vi "Index Texture.vi"(10 "Texture":T1, 11 "Point In Texture":T3) -> (3 "Colour":u32(colorbox))   [LabVIEW 2020, in "Raster (FPGA).lvlib"]
uses:
  Raster (FPGA).lvlib
  Point 2D (I32).ctl
  Texture.ctl
  Rectangle Dimensions.ctl
panel:
  in  "Use Texture (T)":bool=TRUE
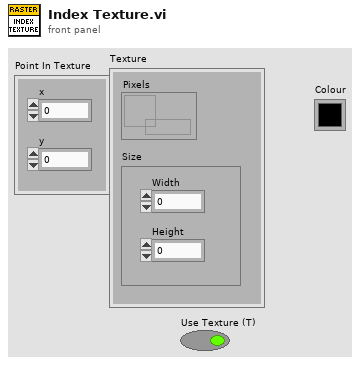
[diagram p1: front panel]
types:
  T1 = typedef "Raster (FPGA).lvlib/Texture.ctl" = cluster{"Pixels":refnum<data-value>, "Size":T2}
  T2 = typedef "Raster (FPGA).lvlib/Rectangle Dimensions.ctl" = cluster{"Width":u32, "Height":u32}
  T3 = typedef "Raster (FPGA).lvlib/Point 2D (I32).ctl" = cluster{"x":i32, "y":i32}
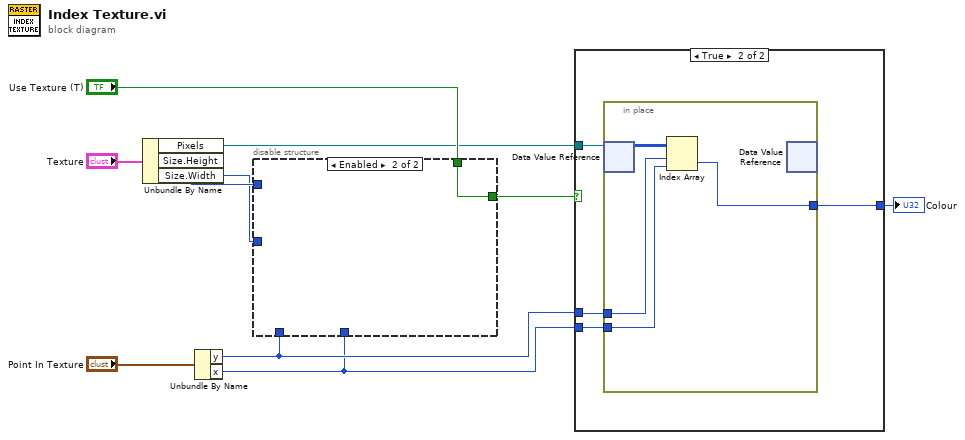
[diagram p0: block diagram]
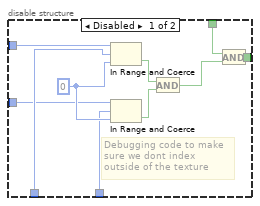
[diagram p2: hidden frame]
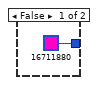
[diagram p3: hidden frame]
diagram:
  n1 = Unbundle By Name("Texture") -> ("Pixels"=w1:refnum<data-value>, "Size.Height"=w4:u32, "Size.Width"=w3:u32)
  n2 = Unbundle By Name("Point In Texture") -> ("y"=w6:i32, "x"=w5:i32)
  n3 = disable-structure shown="Enabled" {
    disable-tunnel: [w17 w21] -> w9
    disable-tunnel: "Use Texture (T)" -> [w15 w21]
    disable-tunnel: w6 -> [w14 _]
    disable-tunnel: w5 -> [w13 _]
    disable-tunnel: w4 -> [w12 _]
    disable-tunnel: w3 -> [w11 _]
    frame Disabled {
      w20 = 0 ("lower limit")
      # "Debugging code to make sure we dont index outside of the texture"
      n4 = In Range and Coerce(upper limit=w12, x=w14, lower limit=w20) -> (In Range?=w19:bool)  [unwired: 1 out]
      n5 = In Range and Coerce(upper limit=w11, x=w13, lower limit=w20) -> (In Range?=w18:bool)  [unwired: 1 out]
      n6 = And(x=w19, y=w18) -> (x .and. y?=w16:bool)
      n7 = And(x=w15, y=w16) -> (x .and. y?=w17:bool)
    }
    frame Enabled {
    }
  }
  n8 = case shown="True" w9 {
    tunnel: w6 -> [_ w25]
    tunnel: w5 -> [_ w24]
    tunnel: [u32 16711880 w23] -> w10
    tunnel: w1 -> [_ w26]
    frame False {
    }
    frame True {
      n9 = in-place {
        in-place-border: w25 -> [w29]
        in-place-border: w24 -> [w28]
        in-place-border: [w27] -> w23
        n10 = in-place-dvr #1(w26) -> (w30:u32[][])  [unwired: 1 out]
        n11 = Index Array(array=w30, index (row)=w29, index (col)=w28) -> (element=w27:u32)
        n12 = in-place-dvr #1() -> ()  [unwired: 1 in, 2 out]
      }
    }
  }
  "Colour" <- w10
